vi "websocket main.vi"(8 "error in":errorcluster, 10 "upgrade data":T1, 11 "websocket handler in":refnum<class "websocket upgrade handler.lvclass">) -> (0 "error out":errorcluster)   [LabVIEW 2016, in "websocket upgrade handler.lvclass"]
uses:
  websocket upgrade handler.lvclass
  HTTP responder/http upgrade data.ctl
  lvlibtls/socket connection/lvlibretls connection.lvclass
  HTTP server/http request.ctl
  HTTP server/http method.ctl
  HTTP headers/http header data.ctl
  websocket upgrade handler.lvclass/websocket upgrade handler.ctl
  user plugin/websocket user plugin.lvclass
  websocket core.lvlib
  HTTP server/Basic HTTPS server.lvclass
  HTTP responder/https responder.lvclass
  HTTP headers/http headers.lvlib
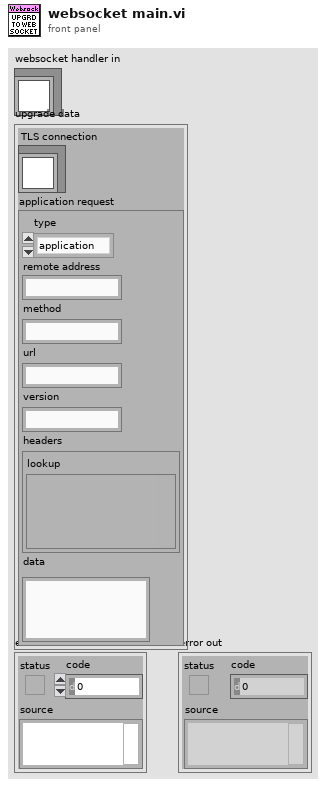
[diagram p1: front panel]
types:
  T1 = typedef "https responder.lvclass/http upgrade data.ctl" = cluster{"TLS connection":refnum<class "lvlibretls connection.lvclass">, "application request":T2}
  T2 = typedef "Basic HTTPS server.lvclass/http request.ctl" = cluster{"type":T3, "remote address":string, "method":string, "url":string, "version":string, "headers":T4, "data":string}
  T3 = typedef "Basic HTTPS server.lvclass/http method.ctl" = enum16{"application", "error", "upgrade"}
  T4 = typedef "http headers.lvlib/http header data.ctl" = cluster{"lookup":variant}
  T5 = typedef "websocket core.lvlib/first byte header.ctl" = cluster{"fin":bool, "RSRV1":bool, "RSRV2":bool, "RSRV3":bool, "opcode":u8}
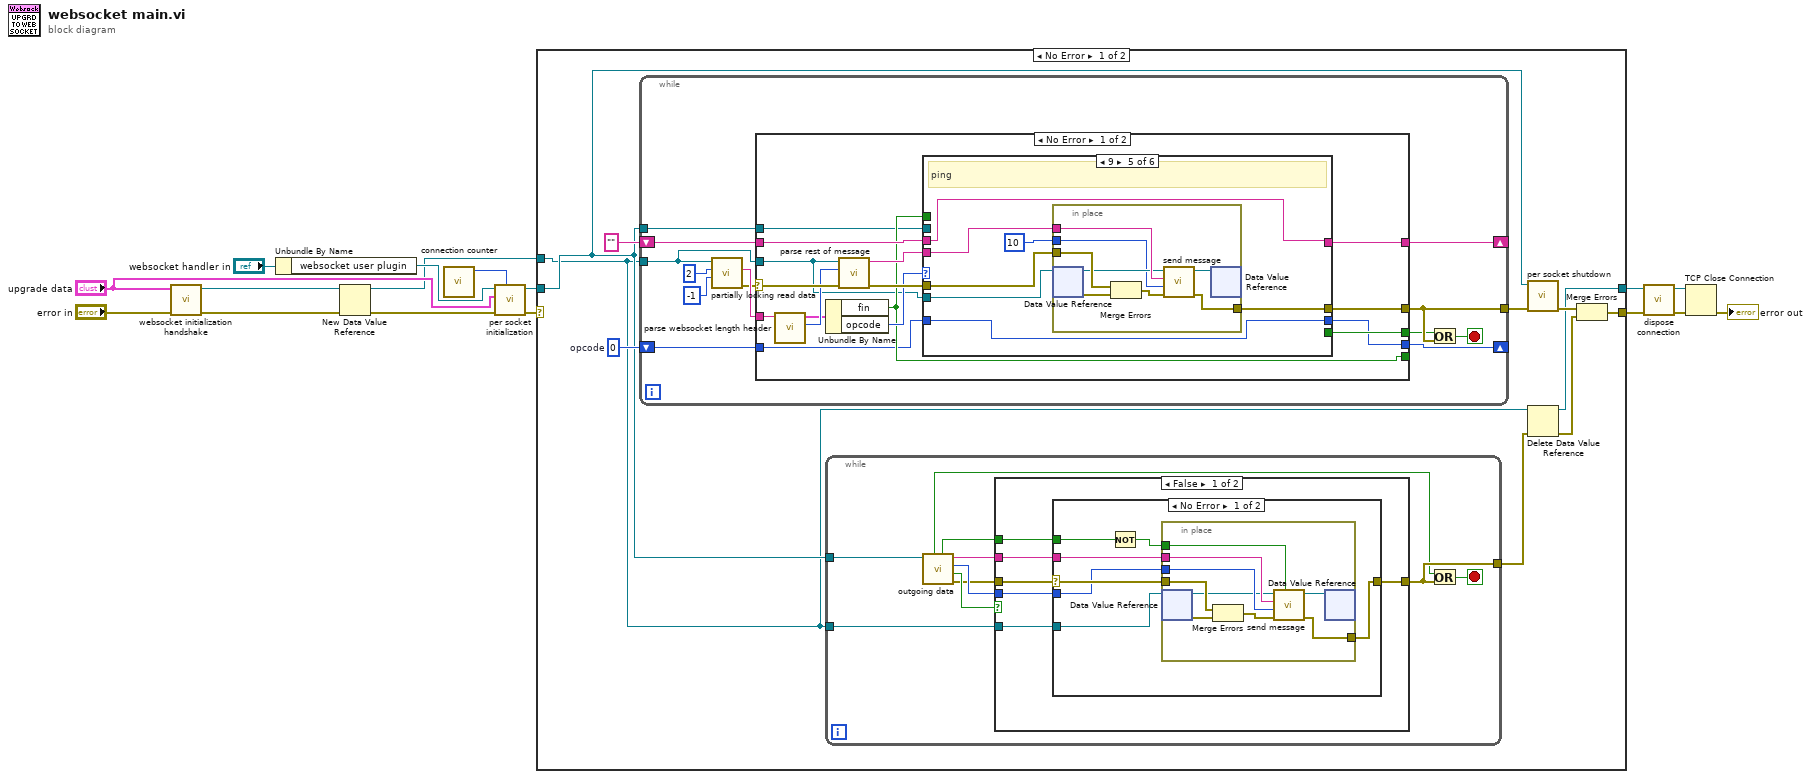
[diagram p0: block diagram]
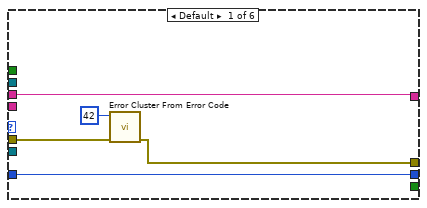
[diagram p4: hidden frame]
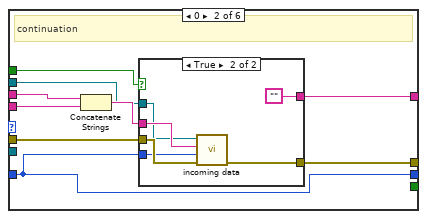
[diagram p5: hidden frame]
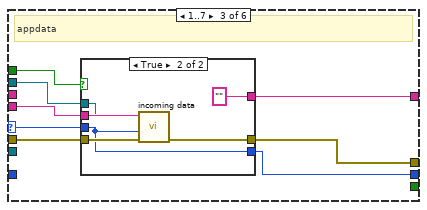
[diagram p7: hidden frame]
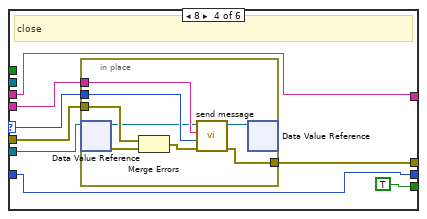
[diagram p9: hidden frame]
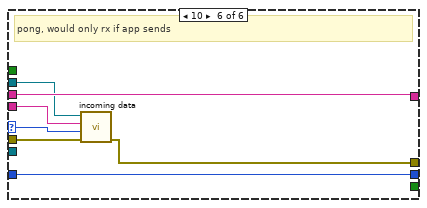
[diagram p10: hidden frame]
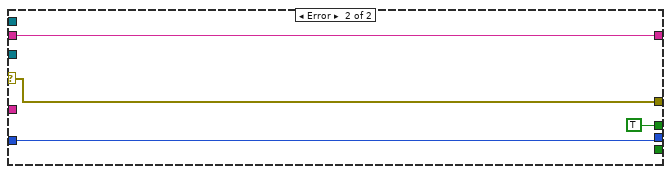
[diagram p11: hidden frame]
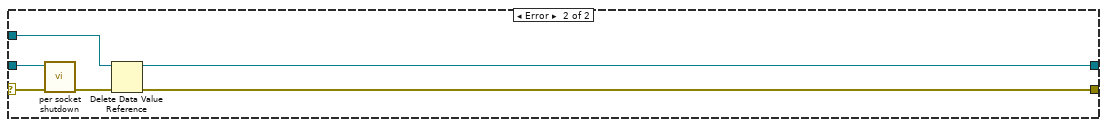
[diagram p12: hidden frame]
diagram:
  n1 = call "websocket initialization handshake.vi"("error in"="error in", "upgrade data"="upgrade data") -> ("error out"=w12:errorcluster, "TLS connection"=w2:refnum<class "lvlibretls connection.lvclass">)  [unwired: 8 in]
  n2 = Unbundle By Name("websocket handler in") -> ("websocket user plugin"=w14:refnum<class "websocket user plugin.lvclass">)
  n3 = New Data Value Reference(data value=w2, error in=w12) -> (data value reference=w1:refnum<data-value>, error out=w3:errorcluster)
  n4 = call "connection counter.vi"() -> ("id"=w9:i32)  [unwired: 11 in]
  n5 = call-dynamic "per socket initialization.vi"("id"=w9, "error in"=w3, "upgrade data"="upgrade data", "websocket user plugin in"=w14) -> ("error out"=w11:errorcluster, "websocket user plugin out"=w13:refnum<class "websocket user plugin.lvclass">)  [unwired: 6 in]
  n6 = case shown="No Error" w11 {
    selector: w11 -> [_ w176]
    tunnel: w1 -> [w17 w172]
    tunnel: [w22 w173] -> w8
    tunnel: w13 -> [w21 w174]
    tunnel: [w18 w171] -> w4
    frame No Error {
      w24 = u8 0  # opcode
      n7 = while {
        tunnel: w17 -> [w61]
        tunnel: [w73] -> w23
        shift-right: [w71] -> _
        shift-left: "" -> [w72]
        shift-right: [w69] -> _
        shift-left: w24 -> [w70]
        tunnel: w21 -> [w68]
        stop <- w67 stop-if-true
        n8 = call "partially locking read data.vi"("timeout"=-1 ("timeout ms (25000)"), "max size"=2 ("bytes to read"), "lvlibretls connection"=w61) -> ("error out"=w62:errorcluster, "data"=w63:string)  [unwired: 7 in]
        n9 = case shown="No Error" w62 {
          selector: w62 -> [w89 w170]
          tunnel: w61 -> [w74 _]
          tunnel: [w86 w170] -> w73
          tunnel: w72 -> [w82 w169]
          tunnel: [w83 w169] -> w71
          tunnel: [w80 _] -> _
          tunnel: w70 -> [w76 w168]
          tunnel: [w77 w168] -> w69
          tunnel: w68 -> [w79 _]
          tunnel: [w78 TRUE] -> w66
          tunnel: w63 -> [w75 _]
          frame No Error {
            n10 = call "parse websocket length header.vi"("header string"=w75) -> ("mask(1)+length(7)"=w88:u8, "first byte"=w87:T5)  [unwired: 9 in]
            n11 = Unbundle By Name(w87) -> ("fin"=w80:bool, "opcode"=w84:u8)
            n12 = call "parse rest of message.vi"("error in"=w89, "mask(1)+length(7)"=w88, "lvlibretls connection in"=w74) -> ("error out"=w85:errorcluster, "unmasked data"=w81:string)  [unwired: 7 in]
            n13 = case shown="9" w84 {
              selector: w84 -> [_ _ w113 w132 _ w160]
              tunnel: [w93 w101 w119 w134 w145 w164] -> w86
              tunnel: w85 -> [w94 w100 w118 w135 w147 w163]
              tunnel: [w91 w97 w115 w131 w151 w166] -> w83
              tunnel: w82 -> [w91 w103 _ w131 w151 w166]
              tunnel: w81 -> [_ w102 w116 w136 w148 w161]
              tunnel: w80 -> [_ w99 w117 _ _ _]
              tunnel: w79 -> [_ w96 w114 _ _ w162]
              tunnel: w74 -> [_ _ _ w129 w146 _]
              tunnel: [_ _ _ TRUE _ _] -> w78
              tunnel: [w90 w95 w112 w130 w150 w165] -> w77
              tunnel: w76 -> [w90 w95 _ w130 w150 w165]
              frame Default {
                n14 = call <vilib>:"Error Cluster From Error Code.vi"("error in (no error)"=w94, "error code (0)"=42) -> ("error out"=w93:errorcluster)  [unwired: 7 in]
              }
              frame 0 {
                # "continuation"
                n15 = Concatenate Strings(w103, w102) -> (w98:string)
                n16 = case shown="True" w99 {
                  tunnel: [w105 w111] -> w101
                  tunnel: w100 -> [w105 w110]
                  tunnel: w98 -> [w104 w109]
                  tunnel: [w104 ""] -> w97
                  tunnel: w96 -> [_ w107]
                  tunnel: w95 -> [_ w106]
                  frame False {
                  }
                  frame True {
                    n17 = call-dynamic "incoming data.vi"("error in"=w110, "opcode"=w106, "data"=w109, "websocket user plugin in"=w107) -> ("error out"=w111:errorcluster)  [unwired: 7 in]
                  }
                }
              }
              frame 1..7 {
                # "appdata"
                n18 = case shown="True" w117 {
                  tunnel: [w122 w128] -> w119
                  tunnel: w118 -> [w122 w127]
                  tunnel: w116 -> [w121 w126]
                  tunnel: [w121 ""] -> w115
                  tunnel: w114 -> [_ w124]
                  tunnel: w113 -> [w120 w123]
                  tunnel: [w120 w123] -> w112
                  frame False {
                  }
                  frame True {
                    n19 = call-dynamic "incoming data.vi"("error in"=w127, "opcode"=w123, "data"=w126, "websocket user plugin in"=w124) -> ("error out"=w128:errorcluster)  [unwired: 7 in]
                  }
                }
              }
              frame 8 {
                # "close"
                n20 = in-place {
                  in-place-border: w136 -> [w144]
                  in-place-border: w135 -> [w143]
                  in-place-border: [w142] -> w134
                  in-place-border: w132 -> [w141]
                  n21 = in-place-dvr #1(w129) -> (w138:refnum<class "lvlibretls connection.lvclass">, w137:errorcluster)
                  n22 = Merge Errors(w143, w137) -> (w140:errorcluster)
                  n23 = call "send message.vi"("error in"=w140, "opcode"=w141, "data"=w144, "lvlibretls connection in"=w138) -> ("error out"=w142:errorcluster, "lvlibretls connection out"=w139:refnum<class "lvlibretls connection.lvclass">)  [unwired: 6 in]
                  n24 = in-place-dvr #1(w139) -> ()  [unwired: 2 out]
                }
              }
              frame 9 {
                # "ping"
                n25 = in-place {
                  in-place-border: w148 -> [w159]
                  in-place-border: w147 -> [w158]
                  in-place-border: [w157] -> w145
                  in-place-border: u8 10 ("opcode") -> [w152]
                  n26 = in-place-dvr #2(w146) -> (w154:refnum<class "lvlibretls connection.lvclass">, w153:errorcluster)
                  n27 = Merge Errors(w158, w153) -> (w156:errorcluster)
                  n28 = call "send message.vi"("error in"=w156, "opcode"=w152, "data"=w159, "lvlibretls connection in"=w154) -> ("error out"=w157:errorcluster, "lvlibretls connection out"=w155:refnum<class "lvlibretls connection.lvclass">)  [unwired: 6 in]
                  n29 = in-place-dvr #2(w155) -> ()  [unwired: 2 out]
                }
              }
              frame 10 {
                # "pong, would only rx if app sends"
                n30 = call-dynamic "incoming data.vi"("error in"=w163, "opcode"=w160, "data"=w161, "websocket user plugin in"=w162) -> ("error out"=w164:errorcluster)  [unwired: 7 in]
              }
            }
          }
          frame Error {
          }
        }
        n31 = Or(x=w66, y=w73) -> (x .or. y?=w67:bool)
      }
      n32 = while {
        tunnel: w17 -> [w36]
        tunnel: [w29] -> w20
        tunnel: w21 -> [w35]
        stop <- w28 stop-if-true
        n33 = call-dynamic "outgoing data.vi"("websocket user plugin in"=w35) -> ("error out"=w30:errorcluster, "timeout"=w31:bool, "opcode"=w32:u8, "data"=w33:string, "not last fragment (F)"=w34:bool, "kill connection"=w27:bool)  [unwired: 5 in]
        n34 = case shown="False" w31 {
          tunnel: w36 -> [w42 _]
          tunnel: [w41 w60] -> w29
          tunnel: w30 -> [w40 w60]
          tunnel: w34 -> [w39 _]
          tunnel: w33 -> [w38 _]
          tunnel: w32 -> [w37 _]
          frame False {
            n35 = case shown="No Error" w40 {
              selector: w40 -> [w48 w59]
              tunnel: [w49 w59] -> w41
              tunnel: w42 -> [w43 _]
              tunnel: w39 -> [w47 _]
              tunnel: w38 -> [w45 _]
              tunnel: w37 -> [w44 _]
              frame No Error {
                n36 = Not(x=w47) -> (.not. x?=w46:bool)
                n37 = in-place {
                  in-place-border: [w58] -> w49
                  in-place-border: w48 -> [w57]
                  in-place-border: w46 -> [w56]
                  in-place-border: w45 -> [w55]
                  in-place-border: w44 -> [w54]
                  n38 = in-place-dvr #3(w43) -> (w53:refnum<class "lvlibretls connection.lvclass">, w50:errorcluster)
                  n39 = Merge Errors(w57, w50) -> (w51:errorcluster)
                  n40 = call "send message.vi"("final fragment (T)"=w56, "error in"=w51, "opcode"=w54, "data"=w55, "lvlibretls connection in"=w53) -> ("error out"=w58:errorcluster, "lvlibretls connection out"=w52:refnum<class "lvlibretls connection.lvclass">)  [unwired: 5 in]
                  n41 = in-place-dvr #3(w52) -> ()  [unwired: 2 out]
                }
              }
              frame Error {
              }
            }
          }
          frame True {
          }
        }
        n42 = Or(x=w27, y=w29) -> (x .or. y?=w28:bool)
      }
      n43 = call-dynamic "per socket shutdown.vi"("error in (no error)"=w23, "websocket user plugin in"=w21) -> ("error out"=w26:errorcluster)  [unwired: 9 in]
      n44 = Delete Data Value Reference(data value reference=w17, error in=w20) -> (data value=w18:refnum<class "lvlibretls connection.lvclass">, error out=w19:errorcluster)
      n45 = Merge Errors(w26, w19) -> (w22:errorcluster)
    }
    frame Error {
      n46 = call-dynamic "per socket shutdown.vi"("error in (no error)"=w176, "websocket user plugin in"=w174) -> ("error out"=w175:errorcluster)  [unwired: 9 in]
      n47 = Delete Data Value Reference(data value reference=w172, error in=w175) -> (data value=w171:refnum<class "lvlibretls connection.lvclass">, error out=w173:errorcluster)
    }
  }
  n48 = call "dispose connection.vi"("error in"=w8, "lvlibretls connection in"=w4) -> ("error out"=w7:errorcluster, "connection"=w5:refnum<k5>)  [unwired: 8 in]
  n49 = TCP Close Connection(connection ID=w5, error in (no error)=w7) -> (error out=→"error out":errorcluster)  [unwired: 1 in, 1 out]
